vi "Is a GUID.vi"(2 "string":string) -> (7 "is a GUID?":bool)   [LabVIEW 2009]
doc: "Returns TRUE if string represents a GUID. Otherwise, this function returns FALSE. Expected pattern: {xxxxxxxx-xxxx-xxxx-xxxx-xxxxxxxxxxxx} where xs are 0-9 or A-F (case-insensitive)."
panel:
  # "[OpenG VI Tags] ***Do Not Remove***"
  # "Is a GUID.vi\n\nReturns TRUE if string represents a GUID. Otherwise, this function returns FALSE.  Expected pattern:  {xxxxxxxx-xxxx-xxxx-xxxx-xxxxxxxxxxxx} where xs are 0-9 or A-F (case-insensitive).\n\nCopyright (c) 2005 MKS Instruments, Inc.  All rights reserved.\nDoug Femec, doug_femec@mksinst.com, IM dafemec\n\nPlease visit http://www.OpenG.org to learn about the\nOpen Source LabVIEW software movement.\n\nThis library is free software; you can redistribute it and/or\nmodify it under the terms of the GNU Lesser General Public\nLicense as published by the Free Software Foundation; either\nversion 2.1 of the License, or (at your option) any later version.\nThis library is distributed in the hope that it will be useful,\nbut WITHOUT ANY WARRANTY; without even the implied warranty of\nMERCHANTABILITY or FITNESS FOR A PARTICULAR PURPOSE. See the GNU\nLesser General Public License for more details.\nYou should have received a copy of the GNU Lesser General Public\nLicense along with this library; if not, write to the Free Software\nFoundation, Inc., 59 Temple Place, Suite 330, Boston, MA 02111-1307 USA"
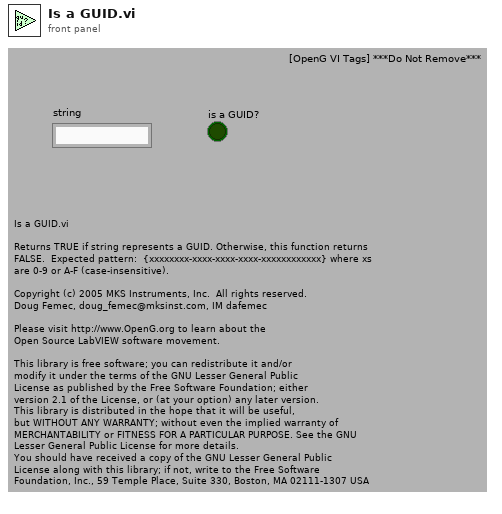
[diagram p1: front panel]
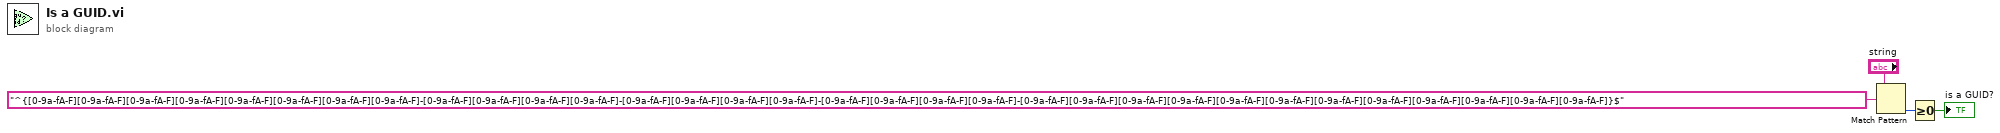
[diagram p0: block diagram]
diagram:
  n1 = Match Pattern(string="string", regular expression="^{[0-9a-fA-F][0-9a-fA-F][0-9a-fA-F][0-9a-fA-F][0-9a-fA-F][0-9a-fA-F][0-9a-fA-F][0-9a-fA-F]-[0-9a-fA-F][0-9a-fA-F][0-9a-fA-F][0-9a-fA-F]-[0-9a-fA-F][0-9a-fA-F][0-9a-fA-F][0-9a-fA-F]-[0-9a-fA-F][0-9a-fA-F][0-9a-fA-F][0-9a-fA-F]-[0-9a-fA-F][0-9a-fA-F][0-9a-fA-F][0-9a-fA-F][0-9a-fA-F][0-9a-fA-F][0-9a-fA-F][0-9a-fA-F][0-9a-fA-F][0-9a-fA-F][0-9a-fA-F][0-9a-fA-F]}$") -> (offset past match=w2:i32)  [unwired: 1 in, 3 out]
  n2 = Greater Or Equal To 0?(x=w2) -> (x >= 0?=→"is a GUID?":bool)
